vi "CRC 异或.vi"(11 "input hex":string) -> (3 "*(类型 *) &x":string)   [LabVIEW 2013]
panel:
  out "无符号字节数组":u8[](array[numeric])
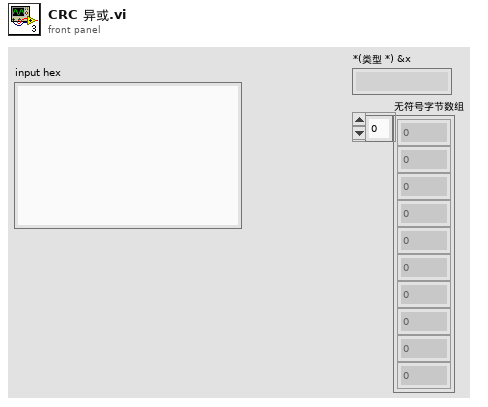
[diagram p1: front panel]
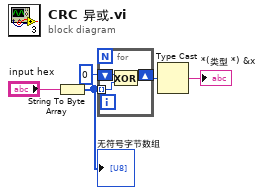
[diagram p0: block diagram]
diagram:
  n1 = String To Byte Array(string="input hex") -> (unsigned byte array=w3:u8[])
  "无符号字节数组" <- w3
  n2 = for {
    tunnel: w3 -> [w8] mode=indexing
    shift-right: [w6] -> w5
    shift-left: u8 0 ("y") -> [w7]
    n3 = Exclusive Or(1:w8, 2:w7) -> (0:w6:u8)
  }
  n4 = Type Cast(x=w5) -> (*(type *) &x=→"*(类型 *) &x":string)  [unwired: 1 in]
